vi "SLMReDisplay.vi"(10 "displayed matrix":u8[][](array[numeric])=array600x792[475200 elements]) -> ()   [LabVIEW 2014]
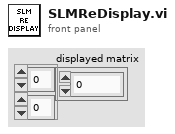
[diagram p1: front panel]
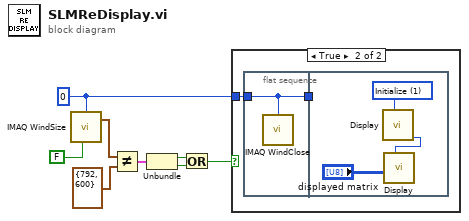
[diagram p0: block diagram]
diagram:
  w1 = 0
  n1 = call "IMAQ WindSize"("Get/Set Status? (Set)"=FALSE, "Window Number"=w1) -> ("Width & Height out"=w3:cluster{"Width":i32, "Height":i32})  [unwired: 3 in, 3 out]
  n2 = Not Equal?(x=w3, y=cluster{"Width":i32, "Height":i32} {"Width"=792, "Height"=600} ("Width & Height out 2")) -> (x != y?=w7:cluster{"Width":bool, "Height":bool})
  n3 = Unbundle(w7) -> ("Width"=w6:bool, "Height"=w5:bool)
  n4 = Or(x=w6, y=w5) -> (x .or. y?=w2:bool)
  n5 = case shown="True" w2 {
    tunnel: w1 -> [_ w10]
    frame False {
    }
    frame True {
      n6 = flat-sequence {
        tunnel: w10 -> [w11]
        tunnel: [w11] -> w9
        tunnel: w9 -> [_]
        frame #0 {
          n7 = call "IMAQ WindClose"("Window Number (0...15)"=w11) -> ()  [unwired: 2 in, 4 out]
        }
        frame #1 {
          w14 = u16 1 items=["Read", "Initialize"] ("Action")
          n8 = call "Display.vi"("Action"=w14) -> ("Read action"=w13:u16)  [unwired: 10 in]
          n9 = call "Display.vi"("Action"=w13, "displayed matrix"="displayed matrix") -> ()  [unwired: 9 in, 1 out]
        }
      }
    }
  }
